vi "FTW-Supervisor-LogEvent.vi"(0 "FTW Supervisor Connection":refnum<class "FTW-Supervisor-Connector.lvclass">, 5 "Event Type":string, 7 "Event Data":string, 9 "Source (unwired for call chain)":string="CallChain", 11 "error in":errorcluster) -> (4 "FTW Supervisor Connection out":refnum<class "FTW-Supervisor-Connector.lvclass">, 15 "error out":errorcluster)   [LabVIEW 2014, in "FTW-Supervisor-Connector.lvclass"]
uses:
  FTW-Supervisor-Connector.lvclass
  connector/FTW-Actor-Connector.lvclass
panel:
  # "Inputs"
  # "Outputs"
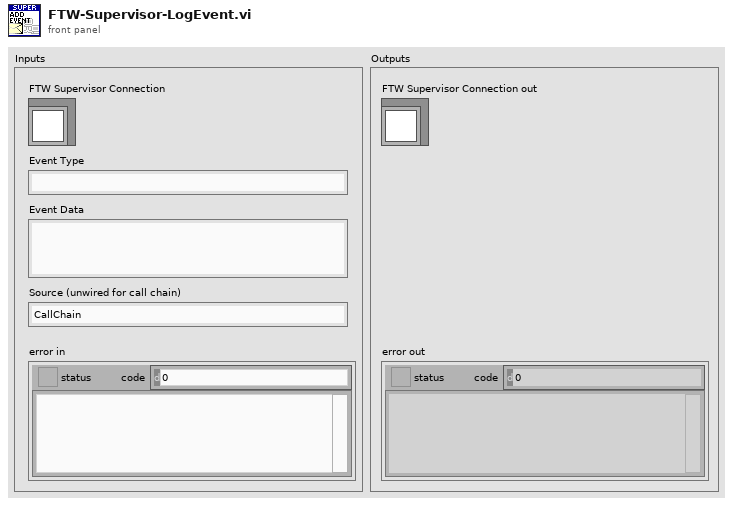
[diagram p1: front panel]
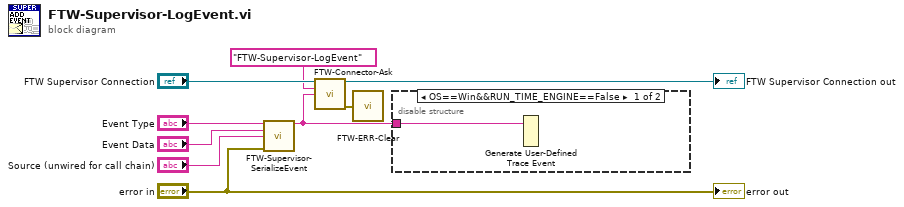
[diagram p0: block diagram]
diagram:
  n1 = call "FTW-Supervisor-SerializeEvent.vi"("Event Type"="Event Type", "Event Data"="Event Data", "Source (unwired for call chain, Empty to omit)"="Source (unwired for call chain)", "Error to Log"="error in") -> ("Serialized Event"=w3:string)  [unwired: 11 in]
  n2 = call "FTW-Connector-Ask.vi"("FTW Actor Connector"="FTW Supervisor Connection", "Request Header"="FTW-Supervisor-LogEvent" ("Parameter"), "Request Body"=w3) -> ("FTW Actor Connector out"=→"FTW Supervisor Connection out":refnum<class "FTW-Supervisor-Connector.lvclass">, "error out"=w2:errorcluster)  [unwired: 9 in, 2 out]
  n3 = call "FTW-ERR-Clear.vi"("error to snuff"=w2) -> ()  [unwired: 1 out]
  n4 = disable-structure shown="OS==Win&&RUN_TIME_ENGINE==False" {
    disable-tunnel: w3 -> [w10 _]
    frame condition #0 (active) {
      n5 = Generate User-Defined Trace Event(2:w10) -> ()  [unwired: 1 in]
    }
    frame condition #1 {
    }
  }
  "error out" <- "error in"
